vi "addNewElement.vi"(6 "firstItem? (F)":bool, 8 "error in (no error)":errorcluster, 9 "prevObjRef":refnum<vi>, 10 "clusterInfo.reference":refnum<vi>, 11 "Short in":refnum<class "Short.lvclass">) -> (0 "error out":errorcluster, 3 "Short out":refnum<class "Short.lvclass">)   [LabVIEW 2016, in "Short.lvclass"]
uses:
  Short.lvclass
  D:/Code/ts_SALLabVIEW/SALTypeGenerator/Elements/Numeric/Numeric.lvclass
  <vilib>/numeric/LVNumericRepresentation.ctl
  Numeric/Numeric.lvclass/Numeric.ctl
  Signed/Signed.lvclass
  Numeric/Numeric.lvclass
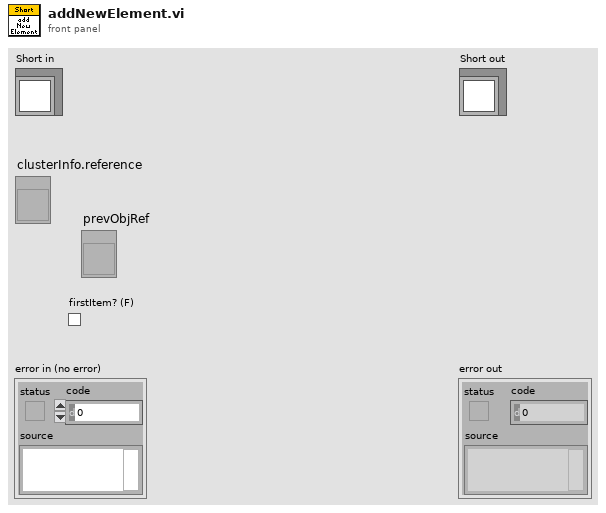
[diagram p1: front panel]
types:
  T1 = typedef "LVNumericRepresentation.ctl" = enum32{"Extended Precision", "Double Precision", "Single Precision", "Long", "Word", "Byte", "Unsigned Long", "Unsigned Word", "Unsigned Byte", "Complex Extended", "Complex Double", "Complex Single", "Quad", "Unsigned Quad", "Fixed-Point"}
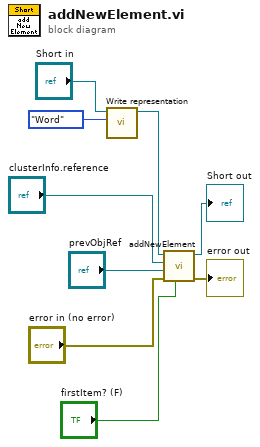
[diagram p0: block diagram]
diagram:
  n1 = call "Write representation.vi"("Numeric Representation"=LVNumericRepresentation."Word", "Numeric in"="Short in") -> ("Numeric out"=w2:refnum<class "Short.lvclass">)  [unwired: 9 in]
  n2 = call-parent "addNewElement.vi"("firstItem? (F)"="firstItem? (F)", "error in (no error)"="error in (no error)", "prevObjRef"="prevObjRef", "clusterInfo.reference"="clusterInfo.reference", "Numeric in"=w2) -> ("error out"=→"error out":errorcluster, "Numeric out"=→"Short out":refnum<class "Short.lvclass">)  [unwired: 5 in]
